vi "Pockels Cal-Ctrl setup.vi"(8 "error in (no error)":errorcluster, 11 "State":T1) -> (0 "error out":errorcluster)   [LabVIEW 2020]
uses:
  Typedefs/Pockels cal wizard states.ctl
  Globals/gl_Calibration globals.vi
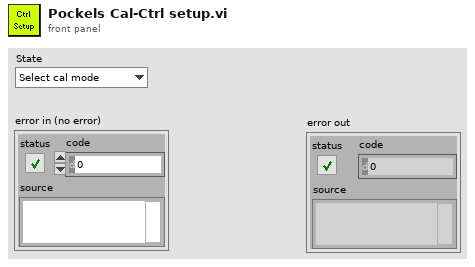
[diagram p1: front panel]
types:
  T1 = typedef "Pockels cal wizard states.ctl" = enum16{"Select cal mode", "Show instructions 1", "Select channel", "Show instructions 2", "Show instructions 3", "Confirm start", "Start calibration"}
  T2 = enum8{"Enabled", "Disabled", "Disabled and Grayed Out"}
  T3 = typedef "Cal mode.ctl" = enum16{"Automatic", "Interactive"}
  T4 = typedef "Pre-AOL Z wizard refs.ctl" = cluster{"VI's reference":refnum<vi>, "Calibration Mode":refnum<vi>, "Cal points":refnum<vi>, "Channel Selector":refnum<vi>, "Message":refnum<vi>, "Back":refnum<vi>, "Next":refnum<vi>, "Power meter AI":refnum<vi>, "2D Picture":refnum<vi>, "Note":refnum<vi>}
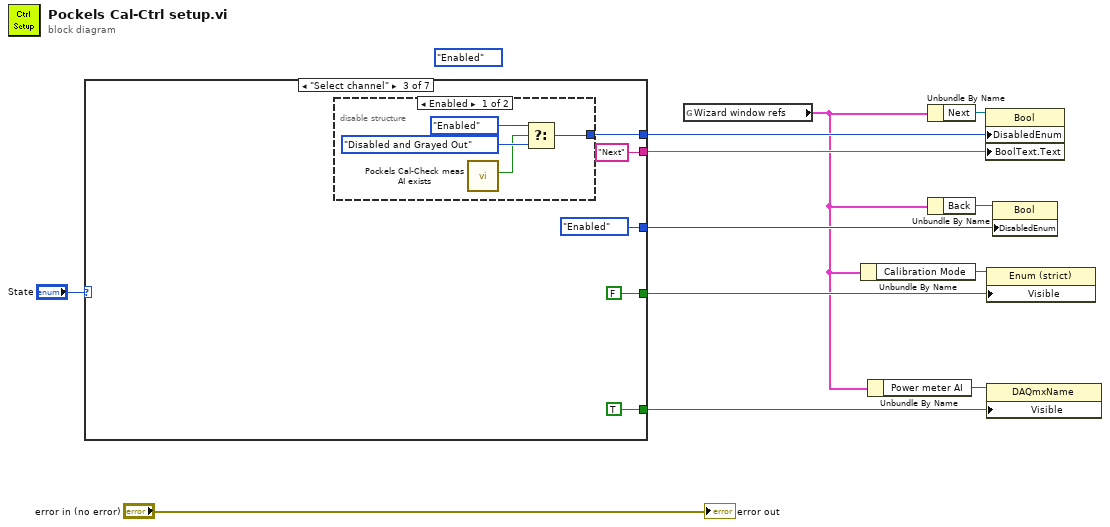
[diagram p0: block diagram]
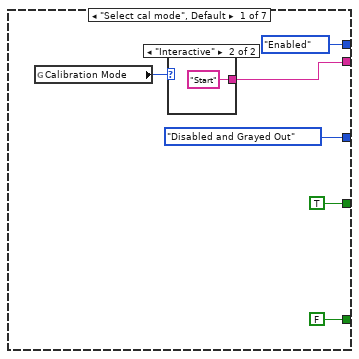
[diagram p2: hidden frame]
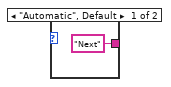
[diagram p3: hidden frame]
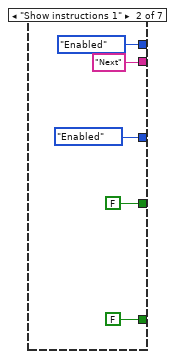
[diagram p4: hidden frame]
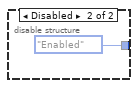
[diagram p5: hidden frame]
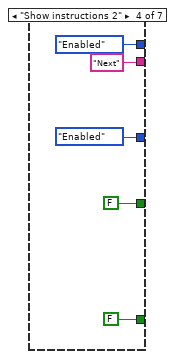
[diagram p6: hidden frame]
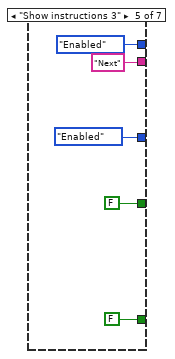
[diagram p7: hidden frame]
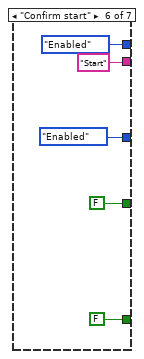
[diagram p8: hidden frame]
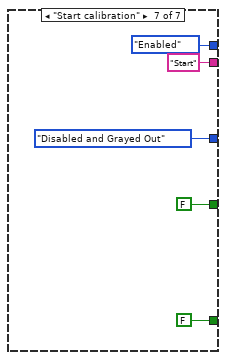
[diagram p9: hidden frame]
diagram:
  (unwired) T2."Enabled" ("Disabled")
  n1 = case shown="\"Select channel\"" "State" {
    tunnel: [TRUE FALSE FALSE FALSE FALSE FALSE FALSE] -> w8
    tunnel: [FALSE FALSE TRUE FALSE FALSE FALSE FALSE] -> w7
    tunnel: [T2."Disabled and Grayed Out" ("Disabled") T2."Enabled" ("Disabled") T2."Enabled" ("Disabled") T2."Enabled" ("Disabled") T2."Enabled" ("Disabled") T2."Enabled" ("Disabled") T2."Disabled and Grayed Out" ("Disabled")] -> w5
    tunnel: [T2."Enabled" ("Disabled") T2."Enabled" ("Disabled") w26 T2."Enabled" ("Disabled") T2."Enabled" ("Disabled") T2."Enabled" ("Disabled") T2."Enabled" ("Disabled")] -> w3
    tunnel: [w13 "Next" ("Boolean Text.Text") "Next" ("Boolean Text.Text") "Next" ("Boolean Text.Text") "Next" ("Boolean Text.Text") "Start" ("Boolean Text.Text") "Start" ("Boolean Text.Text")] -> w2
    frame "Select cal mode", Default {
      n2 = global read "gl_Calibration globals.vi" "Calibration Mode"() -> (w14:T3)
      n3 = case shown="\"Interactive\"" w14 {
        tunnel: ["Next" ("Boolean Text.Text") "Start" ("Boolean Text.Text")] -> w13
        frame "Automatic", Default {
        }
        frame "Interactive" {
        }
      }
    }
    frame "Show instructions 1" {
    }
    frame "Select channel" {
      n4 = disable-structure shown="Enabled" {
        disable-tunnel: [w33 T2."Enabled" ("Disabled")] -> w26
        frame Enabled {
          n5 = call "Pockels Cal-Check meas AI exists.vi"() -> ("Power-meter meas. AI channel exists"=w31:bool)  [unwired: 9 in, 2 out]
          n6 = Select(t=T2."Enabled" ("Disabled"), s=w31, f=T2."Disabled and Grayed Out" ("Disabled")) -> (s? t:f=w33:T2)
        }
        frame Disabled {
        }
      }
    }
    frame "Show instructions 2" {
    }
    frame "Show instructions 3" {
    }
    frame "Confirm start" {
    }
    frame "Start calibration" {
    }
  }
  n7 = global read "gl_Calibration globals.vi" "Wizard window refs"() -> (w1:T4)
  n8 = Unbundle By Name(w1) -> ("Calibration Mode"=w9:refnum<vi>)
  n9 = Unbundle By Name(w1) -> ("Power meter AI"=w10:refnum<vi>)
  n10 = Unbundle By Name(w1) -> ("Next"=w4:refnum<vi>)
  n11 = Unbundle By Name(w1) -> ("Back"=w6:refnum<vi>)
  n12 = property on="Property Node" class="Bool"(reference=w4, "DisabledEnum"=w3, "BoolText.Text"=w2) -> ()  [unwired: 1 in, 2 out]
  n13 = property on="Property Node" class="Enum (strict)"(reference=w9, "Visible"=w8) -> ()  [unwired: 1 in, 2 out]
  n14 = property on="Property Node" class="DAQmxName"(reference=w10, "Visible"=w7) -> ()  [unwired: 1 in, 2 out]
  n15 = property on="Property Node" class="Bool"(reference=w6, "DisabledEnum"=w5) -> ()  [unwired: 1 in, 2 out]
  "error out" <- "error in (no error)"
